vi "ParseSwitch.vi"(7 "Enum":enum16{"Parse", "Convert to string"}(ring)=enum."Convert to string", 9 "cluster in":cluster{"x":dbl, "y":dbl, "z":dbl}, 11 "String":string) -> (1 "pos":string, 3 "output cluster":cluster{"x":dbl, "y":dbl, "z":dbl})   [LabVIEW 2014]
panel:
  out "z":i32
  out "y":i32
  out "x":i32
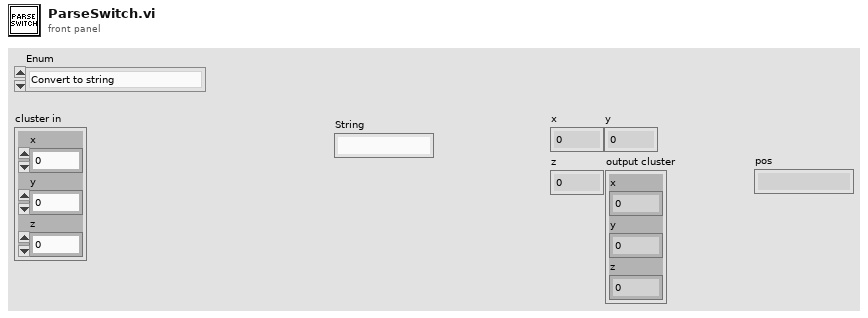
[diagram p1: front panel]
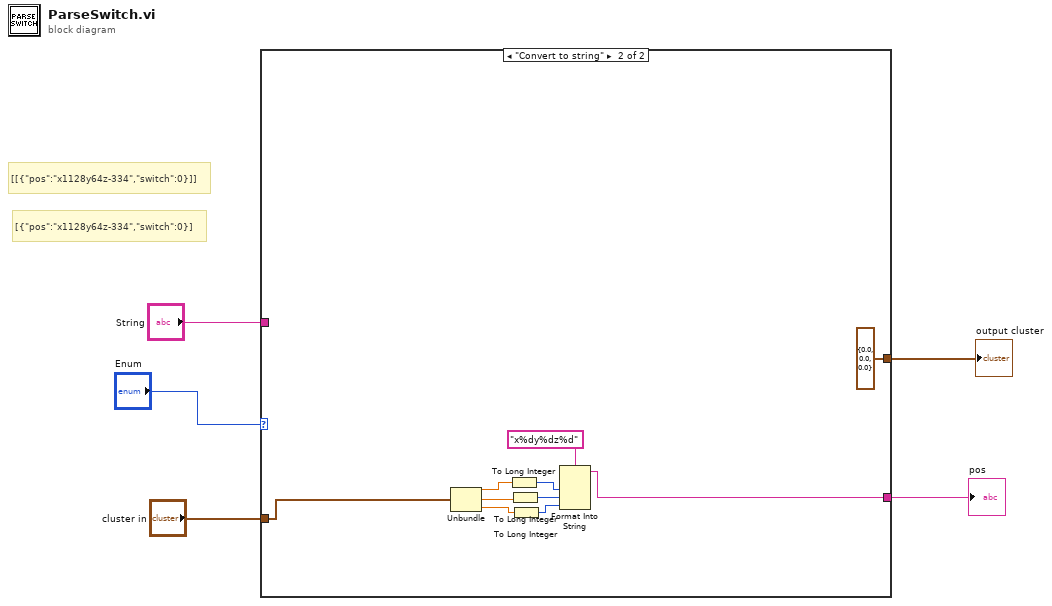
[diagram p0: block diagram]
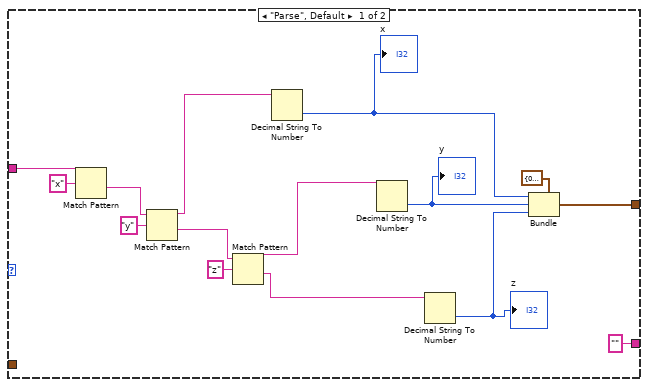
[diagram p2: hidden frame]
diagram:
  # "[{\"pos\":\"x1128y64z-334\",\"switch\":0}]"
  # "[[{\"pos\":\"x1128y64z-334\",\"switch\":0}]]"
  n1 = case shown="\"Convert to string\"" "Enum" {
    tunnel: "String" -> [w20 _]
    tunnel: [w7 cluster{"x":dbl, "y":dbl, "z":dbl} {"x"=0.0, "y"=0.0, "z"=0.0} ("switch_posit")] -> w4
    tunnel: ["" w29] -> w2
    tunnel: "cluster in" -> [_ w30]
    frame "Parse", Default {
      n2 = Match Pattern(string=w20, regular expression="x") -> (after substring=w16:string)  [unwired: 1 in, 3 out]
      n3 = Match Pattern(string=w16, regular expression="y") -> (before substring=w13:string, after substring=w15:string)  [unwired: 1 in, 2 out]
      n4 = Match Pattern(string=w15, regular expression="z") -> (before substring=w12:string, after substring=w14:string)  [unwired: 1 in, 2 out]
      n5 = Decimal String To Number(string=w13) -> (number=w10:i32)  [unwired: 2 in, 1 out]
      "x" <- w10
      n6 = Decimal String To Number(string=w12) -> (number=w9:i32)  [unwired: 2 in, 1 out]
      "y" <- w9
      n7 = Decimal String To Number(string=w14) -> (number=w8:i32)  [unwired: 2 in, 1 out]
      "z" <- w8
      n8 = Bundle(cluster=cluster{"x":dbl, "y":dbl, "z":dbl} {"x"=0.0, "y"=0.0, "z"=0.0} ("switch_posit"), "x"=w10, "y"=w9, "z"=w8) -> (w7:cluster{"x":dbl, "y":dbl, "z":dbl})
    }
    frame "Convert to string" {
      n9 = Unbundle(w30) -> ("x"=w27:dbl, "y"=w22:dbl, "z"=w23:dbl)
      n10 = To Long Integer(number=w27) -> (32bit integer=w26:i32)
      n11 = To Long Integer(number=w22) -> (32bit integer=w21:i32)
      n12 = To Long Integer(number=w23) -> (32bit integer=w24:i32)
      n13 = Format Into String(format string="x%dy%dz%d", w26, w21, w24) -> (resulting string=w29:string)  [unwired: 2 in, 1 out]
    }
  }
  "output cluster" <- w4
  "pos" <- w2
